vi "calculate_smooth_line.vi"(8 "error in (no error)":errorcluster, 11 "TrajectoryDL121017Hopping in":refnum<class "TrajectoryDL121017Hopping.lvclass">) -> (0 "error out":errorcluster, 2 "number of pixels":i32, 3 "TrajectoryDL121017Hopping out":refnum<class "TrajectoryDL121017Hopping.lvclass">)   [LabVIEW 2010, in "TrajectoryDL121017Hopping.lvclass"]
uses:
  TrajectoryDL121017Hopping.lvclass
  segment_cluster.ctl
  common/classes/SpaceVector/SpaceVector/SpaceVector.lvclass
  TrajectoryDL121017Hopping.lvclass/TrajectoryDL121017Hopping.ctl
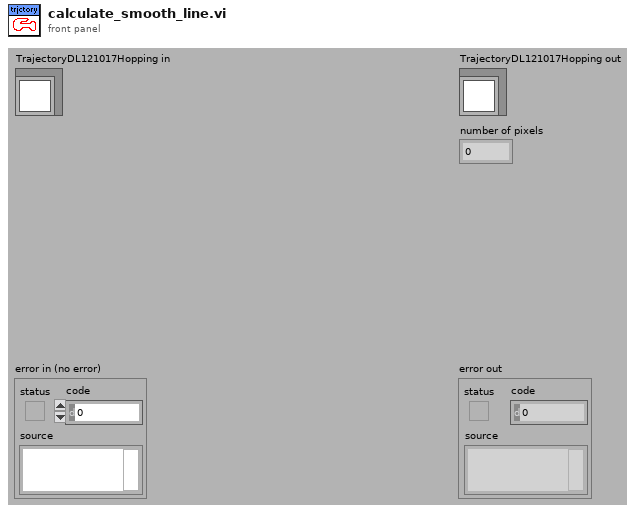
[diagram p1: front panel]
types:
  T1 = typedef "TrajectoryDL121017Hopping.lvclass/segment_cluster.ctl" = cluster{"points":refnum<class "SpaceVector.lvclass">[]}
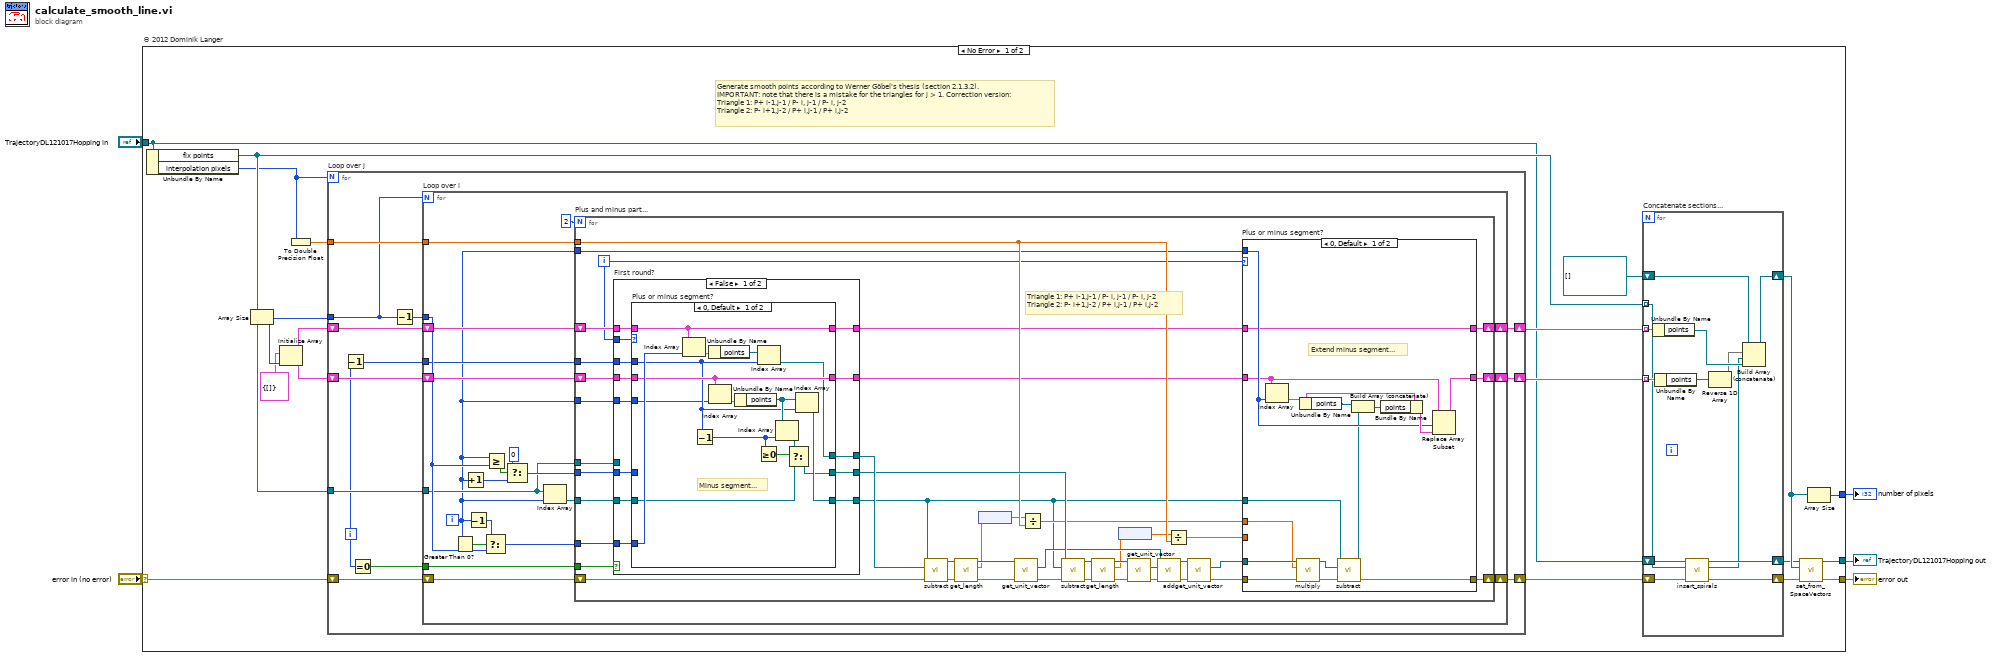
[diagram p0: block diagram]
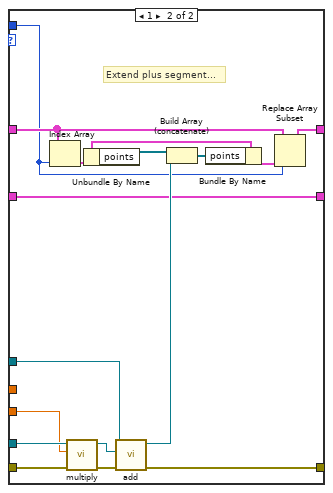
[diagram p2: hidden frame]
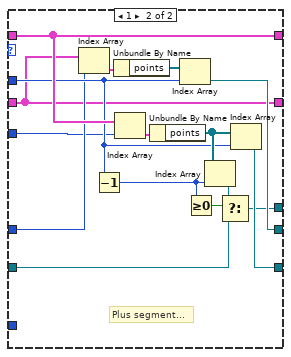
[diagram p3: hidden frame]
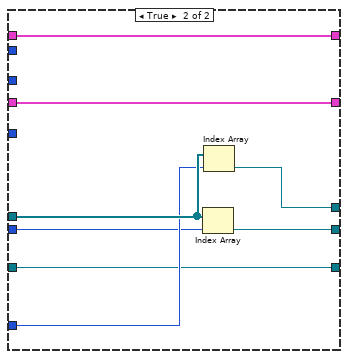
[diagram p4: hidden frame]
diagram:
  n1 = case "© 2012 Dominik Langer" shown="No Error" "error in (no error)" {
    selector: "error in (no error)" -> [w23 w199]
    tunnel: "TrajectoryDL121017Hopping in" -> [w9 w200]
    tunnel: [w15 w199] -> w1
    tunnel: [w16 w200] -> w2
    tunnel: [w12 _] -> w3
    frame No Error {
      # "Generate smooth points according to Werner Göbel's thesis (section 2.1.3.2). \nIMPORTANT: note that there is a mistake for the triangles for j > 1. Correction version:\nTriangle 1: P+ i-1,j-1 / P- i, j-1 / P- i, j-2\nTriangle 2: P- i+1,j-2 / P+ i,j-1 / P+ i,j-2"
      n2 = Unbundle By Name(w9) -> ("fix points"=w17:refnum<class "SpaceVector.lvclass">[], "interpolation pixels"=w10:i32)
      n3 = Array Size(array=w17) -> (size(s)=w20:i32)
      n4 = Initialize Array(T1 {"points"=[]} ("segment"), w20) -> (w19:T1[])
      n5 = To Double Precision Float(number=w10) -> (double precision float=w22:dbl)
      n6 = for "Loop over j" {
        N: w10 -> [_]
        tunnel: w17 -> [w47]
        shift-right: [w48] -> w8
        shift-left: w23 -> [w49]
        shift-right: [w45] -> w21
        shift-left: w19 -> [w46]
        shift-right: [w43] -> w14
        shift-left: w19 -> [w44]
        tunnel: w22 -> [w42]
        tunnel: w20 -> [w38]
        i -> [w40]
        n7 = Decrement(x=w40) -> (x-1=w41:i32)
        n8 = Equal To 0?(x=w40) -> (x = 0?=w39:bool)
        n9 = Decrement(x=w38) -> (x-1=w37:i32)
        n10 = for "Loop over i" {
          N: w38 -> [_]
          shift-right: [w68] -> w48
          shift-left: w49 -> [w70]
          tunnel: w47 -> [w53]
          shift-right: [w66] -> w45
          shift-left: w46 -> [w59]
          shift-right: [w67] -> w43
          shift-left: w44 -> [w57]
          tunnel: w42 -> [w69]
          tunnel: w37 -> [w56]
          tunnel: w41 -> [w54]
          tunnel: w39 -> [w52]
          i -> [w50]
          n11 = Greater Than 0?(x=w50) -> (x > 0?=w65:bool)
          n12 = Increment(x=w50) -> (x+1=w60:i32)
          n13 = Decrement(x=w50) -> (x-1=w64:i32)
          n14 = Select(t=w64, s=w65, f=w56) -> (s? t:f=w58:i32)
          n15 = Greater Or Equal?(x=w50, y=w56) -> (x >= y?=w63:bool)
          n16 = Select(t=0, s=w63, f=w60) -> (s? t:f=w62:i32)
          n17 = Index Array(array=w53, index=w50) -> (element=w55:refnum<class "SpaceVector.lvclass">)
          n18 = for "Plus and minus part..." {
            N: 2 -> [_]
            tunnel: w69 -> [w95]
            tunnel: w62 -> [w84]
            tunnel: w50 -> [w73]
            tunnel: w58 -> [w82]
            tunnel: w55 -> [w80]
            tunnel: w54 -> [w79]
            tunnel: w53 -> [w78]
            tunnel: w52 -> [w77]
            shift-right: [w85] -> w66
            shift-left: w59 -> [w83]
            shift-right: [w86] -> w67
            shift-left: w57 -> [w81]
            shift-right: [w87] -> w68
            shift-left: w70 -> [w111]
            tunnel: w50 -> [w72]
            i -> [w71]
            # "Triangle 1: P+ i-1,j-1 / P- i, j-1 / P- i, j-2\nTriangle 2: P- i+1,j-2 / P+ i,j-1 / P+ i,j-2"
            n19 = case "First round?" shown="False" w77 {
              tunnel: [w151 w194] -> w113
              tunnel: [w153 w195] -> w112
              tunnel: w84 -> [w149 w196]
              tunnel: w83 -> [w155 w192]
              tunnel: w82 -> [w158 w197]
              tunnel: w81 -> [w154 w191]
              tunnel: w80 -> [w157 w193]
              tunnel: w79 -> [w156 _]
              tunnel: w78 -> [_ w198]
              tunnel: [w152 w193] -> w76
              tunnel: [w147 w192] -> w75
              tunnel: [w146 w191] -> w74
              tunnel: w71 -> [w150 _]
              tunnel: w72 -> [w148 _]
              frame False {
                n20 = case "Plus or minus segment?" shown="0, Default" w150 {
                  tunnel: w158 -> [w167 _]
                  tunnel: w157 -> [w166 w182]
                  tunnel: w156 -> [w164 w181]
                  tunnel: w155 -> [w163 w190]
                  tunnel: w154 -> [w165 w175]
                  tunnel: [w160 w180] -> w153
                  tunnel: [w162 w179] -> w152
                  tunnel: [w159 w178] -> w151
                  tunnel: w149 -> [_ w177]
                  tunnel: w148 -> [w161 w176]
                  tunnel: [w163 w190] -> w147
                  tunnel: [w165 w175] -> w146
                  frame 0, Default {
                    # "Minus segment..."
                    n21 = Index Array(array=w163, index=w167) -> (element=w174:T1)
                    n22 = Decrement(x=w164) -> (x-1=w170:i32)
                    n23 = Unbundle By Name(w174) -> ("points"=w173:refnum<class "SpaceVector.lvclass">[])
                    n24 = Index Array(array=w165, index=w161) -> (element=w172:T1)
                    n25 = Unbundle By Name(w172) -> ("points"=w171:refnum<class "SpaceVector.lvclass">[])
                    n26 = Index Array(array=w173, index=w164) -> (element=w159:refnum<class "SpaceVector.lvclass">)
                    n27 = Greater Or Equal To 0?(x=w170) -> (x >= 0?=w169:bool)
                    n28 = Index Array(array=w171, index=w170) -> (element=w168:refnum<class "SpaceVector.lvclass">)
                    n29 = Select(t=w168, s=w169, f=w166) -> (s? t:f=w160:refnum<class "SpaceVector.lvclass">)
                    n30 = Index Array(array=w171, index=w164) -> (element=w162:refnum<class "SpaceVector.lvclass">)
                  }
                  frame 1 {
                    # "Plus segment..."
                    n31 = Index Array(array=w175, index=w177) -> (element=w189:T1)
                    n32 = Decrement(x=w181) -> (x-1=w185:i32)
                    n33 = Unbundle By Name(w189) -> ("points"=w188:refnum<class "SpaceVector.lvclass">[])
                    n34 = Index Array(array=w190, index=w176) -> (element=w187:T1)
                    n35 = Unbundle By Name(w187) -> ("points"=w186:refnum<class "SpaceVector.lvclass">[])
                    n36 = Index Array(array=w188, index=w181) -> (element=w180:refnum<class "SpaceVector.lvclass">)
                    n37 = Greater Or Equal To 0?(x=w185) -> (x >= 0?=w184:bool)
                    n38 = Index Array(array=w186, index=w185) -> (element=w183:refnum<class "SpaceVector.lvclass">)
                    n39 = Select(t=w183, s=w184, f=w182) -> (s? t:f=w178:refnum<class "SpaceVector.lvclass">)
                    n40 = Index Array(array=w186, index=w181) -> (element=w179:refnum<class "SpaceVector.lvclass">)
                  }
                }
              }
              frame True {
                n41 = Index Array(array=w198, index=w196) -> (element=w195:refnum<class "SpaceVector.lvclass">)
                n42 = Index Array(array=w198, index=w197) -> (element=w194:refnum<class "SpaceVector.lvclass">)
              }
            }
            n43 = call "subtract.vi"("error in (no error)"=w111, "subtrahend"=w113, "SpaceVector in"=w76) -> ("error out"=w103:errorcluster, "SpaceVector out"=w104:refnum<class "SpaceVector.lvclass">)  [unwired: 7 in]
            n44 = call "get_length.vi"("error in (no error)"=w103, "SpaceVector in"=w104) -> ("error out"=w102:errorcluster, "length"=w96:dbl[unit], "SpaceVector out"=w101:refnum<class "SpaceVector.lvclass">)  [unwired: 7 in]
            n45 = node(w96) -> (w92:dbl)
            n46 = call "get_unit_vector.vi"("error in (no error)"=w102, "SpaceVector in"=w101) -> ("error out"=w110:errorcluster, "unit vector"=w108:refnum<class "SpaceVector.lvclass">)  [unwired: 7 in, 1 out]
            n47 = Divide(x=w92, y=w95) -> (x/y=w93:dbl)
            n48 = call "subtract.vi"("error in (no error)"=w110, "subtrahend"=w76, "SpaceVector in"=w112) -> ("error out"=w98:errorcluster, "SpaceVector out"=w100:refnum<class "SpaceVector.lvclass">)  [unwired: 7 in]
            n49 = call "get_length.vi"("error in (no error)"=w98, "SpaceVector in"=w100) -> ("error out"=w97:errorcluster, "length"=w91:dbl[unit], "SpaceVector out"=w99:refnum<class "SpaceVector.lvclass">)  [unwired: 7 in]
            n50 = node(w91) -> (w90:dbl)
            n51 = call "get_unit_vector.vi"("error in (no error)"=w97, "SpaceVector in"=w99) -> ("error out"=w107:errorcluster, "unit vector"=w109:refnum<class "SpaceVector.lvclass">)  [unwired: 7 in, 1 out]
            n52 = call "add.vi"("error in (no error)"=w107, "vector to be added"=w109, "SpaceVector in"=w108) -> ("error out"=w105:errorcluster, "SpaceVector out"=w106:refnum<class "SpaceVector.lvclass">)  [unwired: 7 in]
            n53 = Divide(x=w90, y=w95) -> (x/y=w88:dbl)
            n54 = call "get_unit_vector.vi"("error in (no error)"=w105, "SpaceVector in"=w106) -> ("error out"=w94:errorcluster, "unit vector"=w89:refnum<class "SpaceVector.lvclass">)  [unwired: 7 in, 1 out]
            n55 = case "Plus or minus segment?" shown="0, Default" w71 {
              tunnel: w94 -> [w121 w130]
              tunnel: w93 -> [w117 _]
              tunnel: w89 -> [w118 w145]
              tunnel: w88 -> [_ w144]
              tunnel: [w119 w141] -> w87
              tunnel: [w125 w131] -> w86
              tunnel: [w123 w138] -> w85
              tunnel: w76 -> [w116 w134]
              tunnel: w75 -> [w123 w133]
              tunnel: w74 -> [w124 w131]
              tunnel: w73 -> [w126 w132]
              frame 0, Default {
                # "Extend minus segment..."
                n56 = Index Array(array=w124, index=w126) -> (element=w129:T1)
                n57 = call "multiply.vi"("error in (no error)"=w121, "factor"=w117, "SpaceVector in"=w118) -> ("error out"=w120:errorcluster, "SpaceVector out"=w122:refnum<class "SpaceVector.lvclass">)  [unwired: 7 in]
                n58 = Unbundle By Name(w129) -> ("points"=w114:refnum<class "SpaceVector.lvclass">[])
                n59 = call "subtract.vi"("error in (no error)"=w120, "subtrahend"=w122, "SpaceVector in"=w116) -> ("error out"=w119:errorcluster, "SpaceVector out"=w115:refnum<class "SpaceVector.lvclass">)  [unwired: 7 in]
                n60 = Build Array (concatenate)(w114, w115) -> (w128:refnum<class "SpaceVector.lvclass">[])
                n61 = Bundle By Name(cluster=w129, "points"=w128) -> (w127:T1)
                n62 = Replace Array Subset(array=w124, new element=w127, index=w126) -> (w125:T1[])
              }
              frame 1 {
                # "Extend plus segment..."
                n63 = Index Array(array=w133, index=w132) -> (element=w137:T1)
                n64 = call "multiply.vi"("error in (no error)"=w130, "factor"=w144, "SpaceVector in"=w145) -> ("error out"=w142:errorcluster, "SpaceVector out"=w143:refnum<class "SpaceVector.lvclass">)  [unwired: 7 in]
                n65 = Unbundle By Name(w137) -> ("points"=w136:refnum<class "SpaceVector.lvclass">[])
                n66 = call "add.vi"("error in (no error)"=w142, "vector to be added"=w143, "SpaceVector in"=w134) -> ("error out"=w141:errorcluster, "SpaceVector out"=w135:refnum<class "SpaceVector.lvclass">)  [unwired: 7 in]
                n67 = Build Array (concatenate)(w136, w135) -> (w139:refnum<class "SpaceVector.lvclass">[])
                n68 = Bundle By Name(cluster=w137, "points"=w139) -> (w140:T1)
                n69 = Replace Array Subset(array=w133, new element=w140, index=w132) -> (w138:T1[])
              }
            }
          }
        }
      }
      n70 = for "Concatenate sections..." {
        tunnel: w17 -> [w25] mode=indexing
        shift-right: [w32] -> w13
        shift-left: refnum<class "SpaceVector.lvclass">[] [] -> [w33]
        tunnel: w21 -> [w36] mode=indexing
        tunnel: w14 -> [w35] mode=indexing
        shift-right: [w27] -> w7
        shift-left: w9 -> [w29]
        shift-right: [w26] -> w6
        shift-left: w8 -> [w28]
        n71 = Unbundle By Name(w36) -> ("points"=w34:refnum<class "SpaceVector.lvclass">[])
        n72 = Unbundle By Name(w35) -> ("points"=w31:refnum<class "SpaceVector.lvclass">[])
        n73 = call "insert_spirals.vi"("error in (no error)"=w28, "SpaceVector in"=w25, "TrajectoryDL121017Hopping in"=w29) -> ("error out"=w26:errorcluster, "fix point with spirals"=w24:refnum<class "SpaceVector.lvclass">[], "TrajectoryDL121017Hopping out"=w27:refnum<class "TrajectoryDL121017Hopping.lvclass">)  [unwired: 6 in]
        n74 = Reverse 1D Array(array=w31) -> (reversed array=w30:refnum<class "SpaceVector.lvclass">[])
        n75 = Build Array (concatenate)(w33, w30, w24, w34) -> (w32:refnum<class "SpaceVector.lvclass">[])
      }
      n76 = call-dynamic "set_from_SpaceVectors.vi"("error in (no error)"=w6, "voxels"=w13, "TrajectoryDL091126GenericVoxel in"=w7) -> ("error out"=w15:errorcluster, "TrajectoryDL091126GenericVoxel out"=w16:refnum<class "TrajectoryDL121017Hopping.lvclass">)  [unwired: 7 in]
      n77 = Array Size(array=w13) -> (size(s)=w12:i32)
    }
    frame Error {
    }
  }
  "error out" <- w1
  "TrajectoryDL121017Hopping out" <- w2
  "number of pixels" <- w3
